vi "cam Resolutions.vi"(8 "error in (no error)":errorcluster, 11 "Camera Selection":string) -> (0 "error out":errorcluster, 2 "Video Modes":T1(array[cluster]), 3 "Refnum out":T2)   [LabVIEW 2024]
uses:
  <vilib>/userDefined/High Color/IMAQdx.ctl
  <vilib>/vision/driver/NI_Vision_Acquisition_Software.lvlib
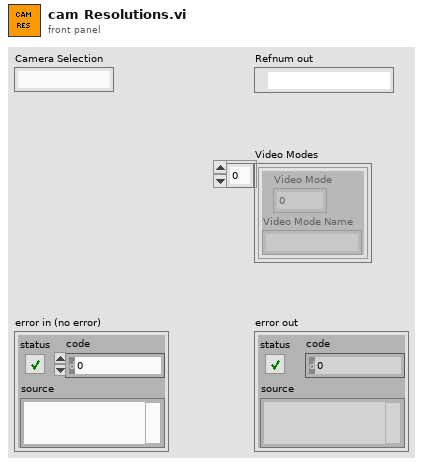
[diagram p1: front panel]
types:
  T1 = cluster{"Video Mode":u32, "Video Mode Name":string}[]
  T2 = typedef "IMAQdx.ctl" = refnum<k21>
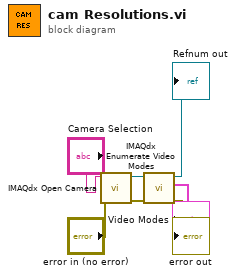
[diagram p0: block diagram]
diagram:
  n1 = call <vilib>:"IMAQdx Open Camera.vi"("error in"="error in (no error)", "Session In"="Camera Selection") -> ("error out"=w3:errorcluster, "Session Out"=w7:T2)  [unwired: 8 in]
  n2 = call <vilib>:"IMAQdx Enumerate Video Modes.vi"("error in"=w3, "Session In"=w7) -> ("error out"=→"error out":errorcluster, "Video Modes"=→"Video Modes":T1, "Session Out"=→"Refnum out":T2)  [unwired: 6 in, 1 out]
